vi "Cache_Hierarchy Load.vi"(8 "error in (no error)":errorcluster, 10 "Class Name":string, 11 "Refnum in":T1) -> (0 "error out":errorcluster, 1 "Success?":bool, 2 "Hierarchy":string[](array[string]), 3 "Refnum out":T1)   [LabVIEW 2019, in "ClassLoader.lvlib"]
uses:
  ClassLoader.lvlib
  <vilib>/Utility/config.llb/NI_LVConfig.lvlib
  <vilib>/Utility/config.llb/Config Data RefNum.ctl
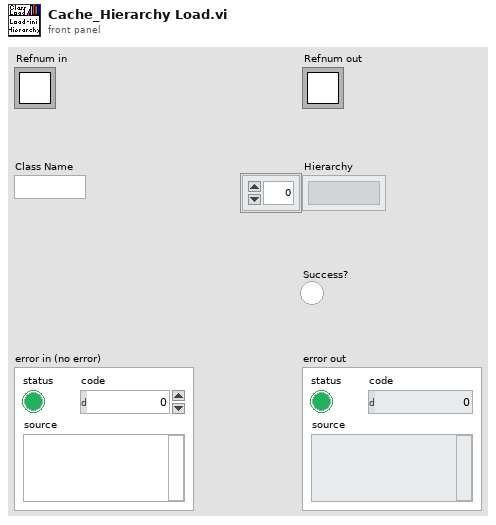
[diagram p1: front panel]
types:
  T1 = typedef "NI_LVConfig.lvlib/Config Data RefNum.ctl" = refnum<k1>
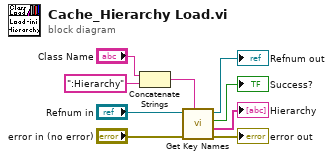
[diagram p0: block diagram]
diagram:
  n1 = Concatenate Strings("Class Name", ":Hierarchy" ("string")) -> (w3:string)
  n2 = call <vilib>:"Get Key Names.vi"("section"=w3, "error in (no error)"="error in (no error)", "refnum"="Refnum in") -> ("error out"=→"error out":errorcluster, "key names"=→"Hierarchy":string[], "section exists?"=→"Success?":bool, "refnum out"=→"Refnum out":T1)  [unwired: 5 in]
